vi "Experiment header-append to Imaging modes.vi"(7 "Header file sections":T1=enum."TIME SERIES", 8 "error in (no error)":errorcluster) -> (0 "error out":errorcluster)   [LabVIEW 2020]
uses:
  Typedefs/Header file sections.ctl
  Typedefs/Header file interface module functions enum.ctl
  Global Variables/General Globals.vi
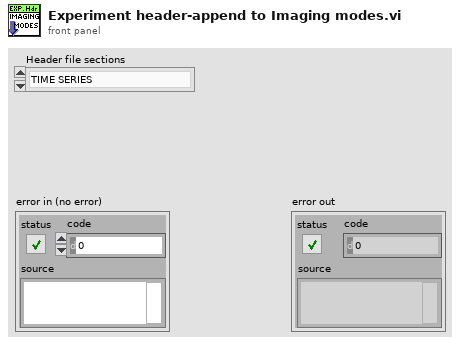
[diagram p1: front panel]
types:
  T1 = typedef "Header file sections.ctl" = enum16{"ALL SECTIONS", "LOGIN", "GLOBAL PARAMETERS", "CALIBRATION DATA", "IMAGING MODES", "TIME SERIES", "MOTOR Z-STACK", "AOL Z-STACK", "FUNCTIONAL IMAGING", "VOLUME IMAGING", "MOVEMENT CORRECTION", "CALIBRATION", "STATISTICS", "BIOLOGY INFORMATION"}
  T2 = typedef "Header file interface module functions enum.ctl" = enum16{"Load experiment header file", "Save experiment header file", "Clear stored values", "Read stored values", "Update specific value in memory", "Update values in memory"}
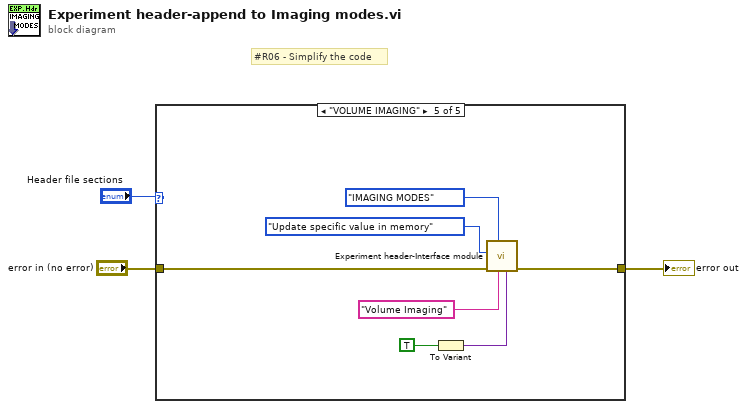
[diagram p0: block diagram]
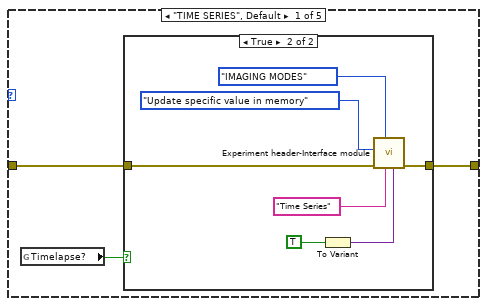
[diagram p2: hidden frame]
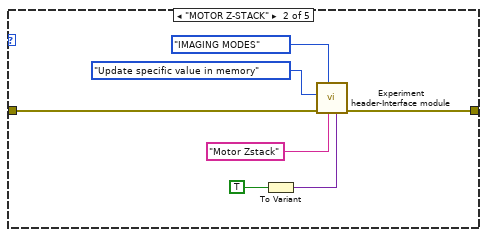
[diagram p4: hidden frame]
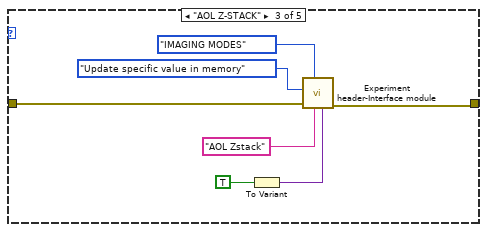
[diagram p5: hidden frame]
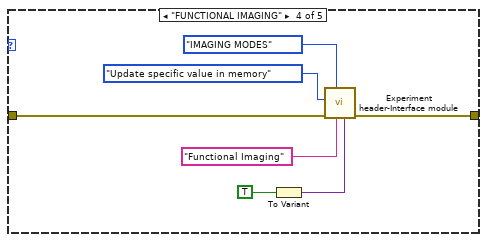
[diagram p6: hidden frame]
diagram:
  # "#R06 - Simplify the code"
  n1 = case shown="\"VOLUME IMAGING\"" "Header file sections" {
    tunnel: "error in (no error)" -> [w5 w16 w23 w30 w37]
    tunnel: [w4 w15 w22 w29 w36] -> w1
    frame "TIME SERIES", Default {
      n2 = global read "General Globals.vi" "Timelapse?"() -> (w6:bool)
      n3 = case shown="True" w6 {
        tunnel: w5 -> [w7 w9]
        tunnel: [w7 w8] -> w4
        frame False {
        }
        frame True {
          n4 = To Variant(anything=TRUE) -> (Variant=w10:variant)
          n5 = call "Experiment header-Interface module.vi"("Value to change"=w10, "Name of parameter to update"="Time Series", "Header file sections"=Header_file_sections."IMAGING MODES", "error in (no error)"=w9, "Function"=Header_file_interface_module_functions_enum."Update specific value in memory") -> ("error out"=w8:errorcluster)  [unwired: 5 in, 1 out]
        }
      }
    }
    frame "MOTOR Z-STACK" {
      n6 = To Variant(anything=TRUE) -> (Variant=w17:variant)
      n7 = call "Experiment header-Interface module.vi"("Value to change"=w17, "Name of parameter to update"="Motor Zstack", "Header file sections"=Header_file_sections."IMAGING MODES", "error in (no error)"=w16, "Function"=Header_file_interface_module_functions_enum."Update specific value in memory") -> ("error out"=w15:errorcluster)  [unwired: 5 in, 1 out]
    }
    frame "AOL Z-STACK" {
      n8 = To Variant(anything=TRUE) -> (Variant=w28:variant)
      n9 = call "Experiment header-Interface module.vi"("Value to change"=w28, "Name of parameter to update"="AOL Zstack", "Header file sections"=Header_file_sections."IMAGING MODES", "error in (no error)"=w23, "Function"=Header_file_interface_module_functions_enum."Update specific value in memory") -> ("error out"=w22:errorcluster)  [unwired: 5 in, 1 out]
    }
    frame "FUNCTIONAL IMAGING" {
      n10 = To Variant(anything=TRUE) -> (Variant=w35:variant)
      n11 = call "Experiment header-Interface module.vi"("Value to change"=w35, "Name of parameter to update"="Functional Imaging", "Header file sections"=Header_file_sections."IMAGING MODES", "error in (no error)"=w30, "Function"=Header_file_interface_module_functions_enum."Update specific value in memory") -> ("error out"=w29:errorcluster)  [unwired: 5 in, 1 out]
    }
    frame "VOLUME IMAGING" {
      n12 = To Variant(anything=TRUE) -> (Variant=w42:variant)
      n13 = call "Experiment header-Interface module.vi"("Value to change"=w42, "Name of parameter to update"="Volume Imaging", "Header file sections"=Header_file_sections."IMAGING MODES", "error in (no error)"=w37, "Function"=Header_file_interface_module_functions_enum."Update specific value in memory") -> ("error out"=w36:errorcluster)  [unwired: 5 in, 1 out]
    }
  }
  "error out" <- w1
